vi "GrabQQ.vi"() -> ()   [LabVIEW 2016]
doc: "The Grab (Express) VI acquires images continuously and displays the images in an image control using the Vision Acquisition Express VI. A grab is appropriate for high-speed applications in which you need to process only one image at a time."
uses:
  <vilib>/Platform/TimedLoop/XDataNode/timing_clust.ctl
  <vilib>/Platform/TimedLoop/XDataNode/nitl_modes.ctl
  <vilib>/Platform/TimedLoop/XDataNode/wakeup.ctl
  <vilib>/platform/TimedLoop/XDataNode/XDataNode.xnode
  <vilib>/Platform/TimedLoop/XDataNode/XDNodeRunTimeDep.lvlib
panel:
  out "Camera":bool
  in  "Manual Stop":bool
  out "Actual interframe (s)":dbl
  in  "Path":path
  in  "Interframe (s)":dbl=1.0
  out "Photo #":i32 caption="iter"
  out "Image":T1(plugin-control)
  in  "Manual Start":bool
  # "Overview: Demonstrates\nRequirements: Vision Acquisition Software\nInstructions: Run the VI"
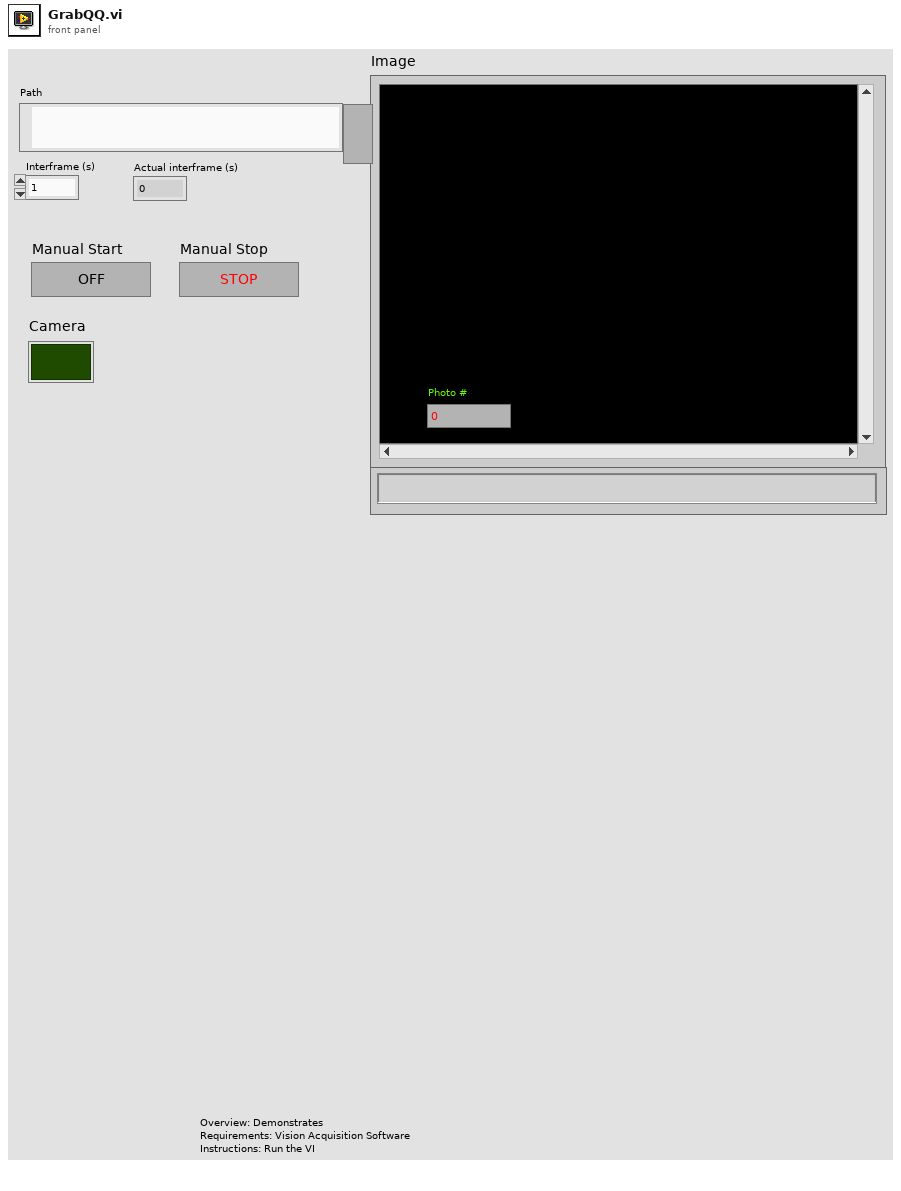
[diagram p1: front panel]
types:
  T1 = typedef "IMAQ Image.ctl" = refnum<image>
  T2 = enum16{"open", "replace", "create", "open or create", "replace or create", "replace or create with confirmation"}
  T3 = typedef "XDNodeRunTimeDep.lvlib/timing_clust.ctl" = cluster{"Expected End [f-1]":u64, "Actual End [f-1]":u64, "Finished Late? [f-1]":bool, "Expected End [i-1]":u64, "Actual End [i-1]":u64, "Finished Late? [i-1]":bool, "Expected Start [i]":u64, "Actual Start [i]":u64, "Expected Start [f]":u64, "Actual Start [f]":u64, "Source Name":string, "Structure Name":string, "Period":i64, "Deadline":i64, "Offset":i64, "Start":i64, "Priority":i32, "Timeout":i32, "Mode":T4, "Wakeup Reason":T5, "Error":errorcluster, "Source Type":string, "Secondary Source Type":string, "Global End Time":u64, "Global Start Time":u64, "Frame Duration":u64, "Iteration Duration":u64, "Assigned CPU":i32, "I/O Scan Engine Mode":u32}
  T4 = typedef "XDNodeRunTimeDep.lvlib/nitl_modes.ctl" = enum32{"No Change", "Process missed periods, maintain original phase", "Discard missed periods, maintain original phase", "Process missed periods, ignore original phase", "Discard missed periods, ignore original phase"}
  T5 = typedef "XDNodeRunTimeDep.lvlib/wakeup.ctl" = enum32{"Normal", "Aborted", "Asynchronous wakeup", "Timing source error", "Timed loop error", "Timeout"}
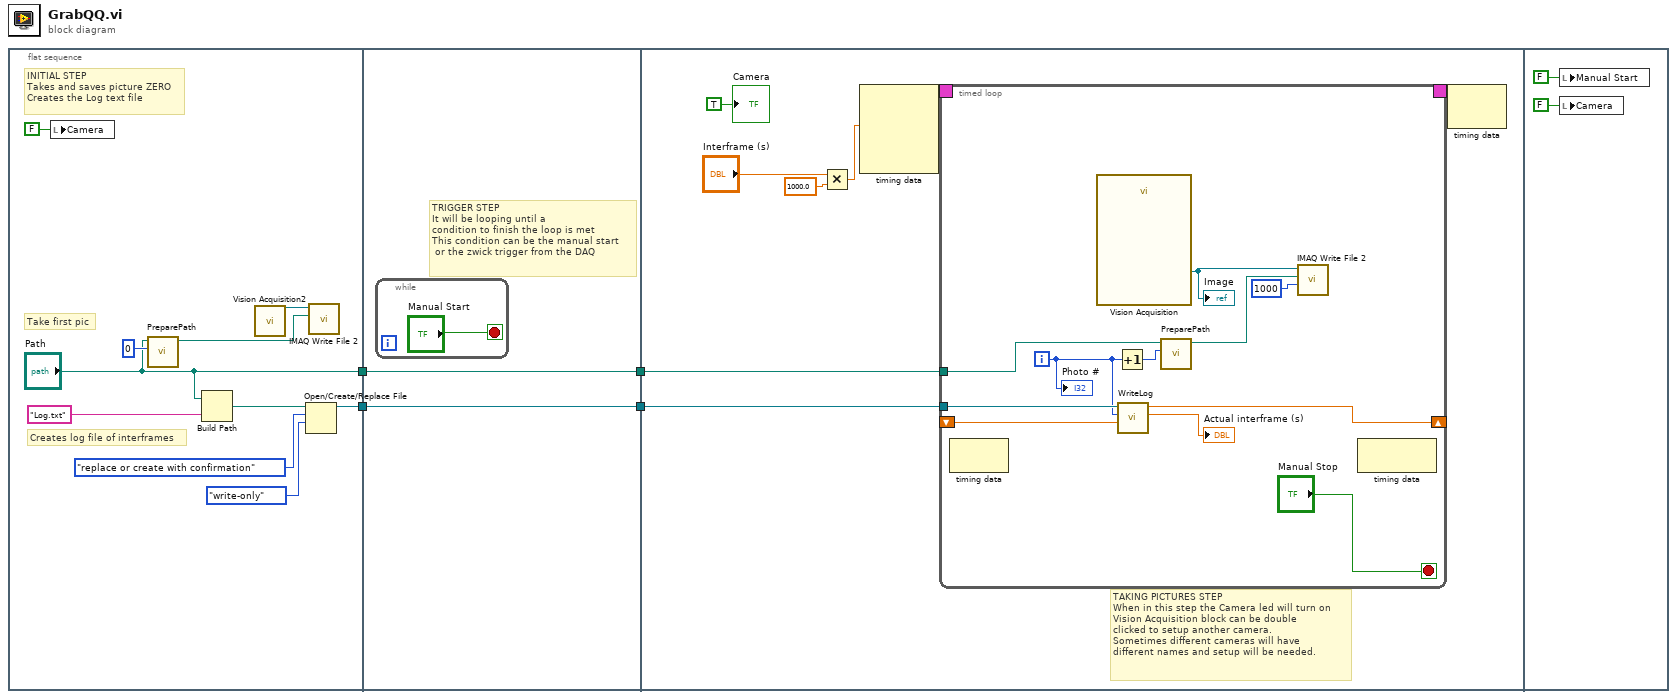
[diagram p0: block diagram]
diagram:
  n1 = flat-sequence {
    tunnel: ["Path"] -> w4
    tunnel: [w9] -> w2
    tunnel: w4 -> [w16]
    tunnel: [w16] -> w3
    tunnel: w2 -> [w15]
    tunnel: [w15] -> w1
    tunnel: w3 -> [w25]
    tunnel: w1 -> [w24]
    frame #0 {
      # "INITIAL STEP\nTakes and saves picture ZERO\nCreates the Log text file"
      # "Creates log file of interframes"
      # "Take first pic"
      n2 = local write "Camera"(FALSE ("Camera")) -> ()
      n3 = call "PreparePath.vi"("Numeric"=0, "Path"="Path") -> ("appended path"=w12:path)  [unwired: 9 in]
      n4 = Build Path(base path="Path", name or relative path="Log.txt") -> (appended path=w5:path)
      n5 = call "Vision Acquisition2"() -> ("Image Out"=w14:T1)  [unwired: 2 in, 25 out]
      n6 = Open/Create/Replace File(file path (use dialog)=w5, operation (0:open)=T2."replace or create with confirmation", access (0:read/write)=enum16{"read/write", "read-only", "write-only"}."write-only") -> (refnum out=w9:refnum<file>)  [unwired: 3 in, 2 out]
      n7 = call-poly "IMAQ Write File 2"("File Path"=w12, "Image"=w14) -> ()  [unwired: 8 in, 2 out]
    }
    frame #1 {
      # "TRIGGER STEP\nIt will be looping until a \ncondition to finish the loop is met\nThis condition can be the manual start\n or the zwick trigger from the DAQ"
      n8 = while {
        stop <- "Manual Start" stop-if-true
      }
    }
    frame #2 {
      # "TAKING PICTURES STEP\nWhen in this step the Camera led will turn on\nVision Acquisition block can be double\nclicked to setup another camera.\nSometimes different cameras will have\ndifferent names and setup will be needed."
      n9 = Multiply(x="Interframe (s)", y=1000.0) -> (x*y=w19:dbl)
      n10 = node-c288(w19) -> (w23:T3)  [unwired: 3 in]
      n11 = timed-loop {
        timing: w23 -> [_]
        timing-out: [_] -> w22
        tunnel: w25 -> [w33]
        shift-right: [w32] -> _
        shift-left: _ -> [w31]
        tunnel: w24 -> [w30]
        i -> [w29]
        stop <- "Manual Stop" stop-if-true
        n12 = node-c288() -> ()  [unwired: 1 in, 1 out]
        n13 = call "Vision Acquisition"() -> ("Image Out"=w35:T1)  [unwired: 2 in, 25 out]
        "Image" <- w35
        n14 = Increment(x=w29) -> (x+1=w34:i32)
        n15 = call "WriteLog.vi"("relative seconds in"=w31, "Numeric"=w29, "Byte Stream File in"=w30) -> ("x-y"=→"Actual interframe (s)":dbl, "relative seconds out"=w32:dbl)  [unwired: 7 in]
        n16 = call "PreparePath.vi"("Numeric"=w34, "Path"=w33) -> ("appended path"=w36:path)  [unwired: 9 in]
        n17 = call-poly "IMAQ Write File 2"("Image Quality"=u32 1000, "File Path"=w36, "Image"=w35) -> ()  [unwired: 7 in, 2 out]
        n18 = node-c288() -> ()  [unwired: 1 in, 1 out]
        "Photo #" <- w29
      }
      n19 = node-c288(w22) -> ()  [unwired: 1 out]
      "Camera" <- TRUE ("Camera")
    }
    frame #3 {
      n20 = local write "Manual Start"(FALSE ("Manual Start")) -> ()
      n21 = local write "Camera"(FALSE ("Camera")) -> ()
    }
  }
